vi "Data_Aquisition_cRIO4.vi"() -> ()   [LabVIEW 2016]
uses:
  <vilib>/Platform/TimedLoop/XDataNode/timing_clust.ctl
  <vilib>/Platform/TimedLoop/XDataNode/nitl_modes.ctl
  <vilib>/Platform/TimedLoop/XDataNode/wakeup.ctl
  <vilib>/Utility/file.llb/Write Delimited Spreadsheet (string).vi
  <vilib>/Platform/TimedLoop/XDataNode/loadnilvce.vi
  <vilib>/Utility/file.llb/Write Delimited Spreadsheet (DBL).vi
  <vilib>/Platform/TimedLoop/XDataNode/XDataNode.xnode
  <vilib>/Platform/TimedLoop/XDataNode/XDNodeRunTimeDep.lvlib
panel:
  in  "Mod 2 Labels":string[][](array[string])=[["M2AO0", "M2AO1"], ["Air", "N2"]]
  in  "Mod 1 Labels":string[][](array[string])=[["M1DO0", "M1DO1", "M1DO2", "M1DO3", "M1DO4", "M1DO5", "M1DO6"], ["Inf", "Eff", "Acid", "Base", "Media", "Air", "Release"]]
  in  "Mod 3 Labels":string[][](array[string])=[["M3AI0", "M3AI1", "M3AI2", "M3AI3", "M3AI4"], ["pH", "DO", "Air", "N2", "Off"]]
  out "data":dbl[][](array[numeric])=[[8.0, 29.0, 2018.0, 14421397.0, 0.0, 0.0, 0.0, 0.0, 0.0, 1.0, 0.0, 0.003999706016, 0.003999847522999999, 0.012958363706999999, 0.004113970148, -1.9721429999999986e-06, 0.0039692390630000005, 0.003999705047], [8.0, 29.0, 2018.0, 14421638.0, 0.0, 0.0, 0.0, 0.0, 0.0, 1.0, 0.0, 0.003999706016, 0.003999847522999999, 0.012891145231999999, 0.004107738319, -1.6440880000000006e-06, 0.003968582989, 0.004000361167]]
  out "headers":string[][](array[string])=[["Month", "Day", "Year", "Time", "M1DO0", "M1DO1", "M1DO2", "M1DO3", "M1DO4", "M1DO5", "M1DO6", "M2DO0", "M2DO1", "M3DO0", "M3DO1", "M3DO2", "M3DO3", "M3DO4"], ["Month", "Day", "Year", "Time", "Inf", "Eff", "Acid", "Base", "Media", "Air", "Release", "Air", "N2", "pH", "DO", "Air", "N2", "Off"]]
  out "Time":string="144216.38"
  out "Date":string="08292018"
  in  "Buffer Size":i32=6
  out "Saving?":bool=TRUE
  out "new file path (Not A Path if cancelled)":path=path "u:/_08292018_140859.csv"
  in  "File Name:":string
  out "error out":errorcluster
  out "iter number":i32=34
  in  "stop":bool
  in  "error in":errorcluster
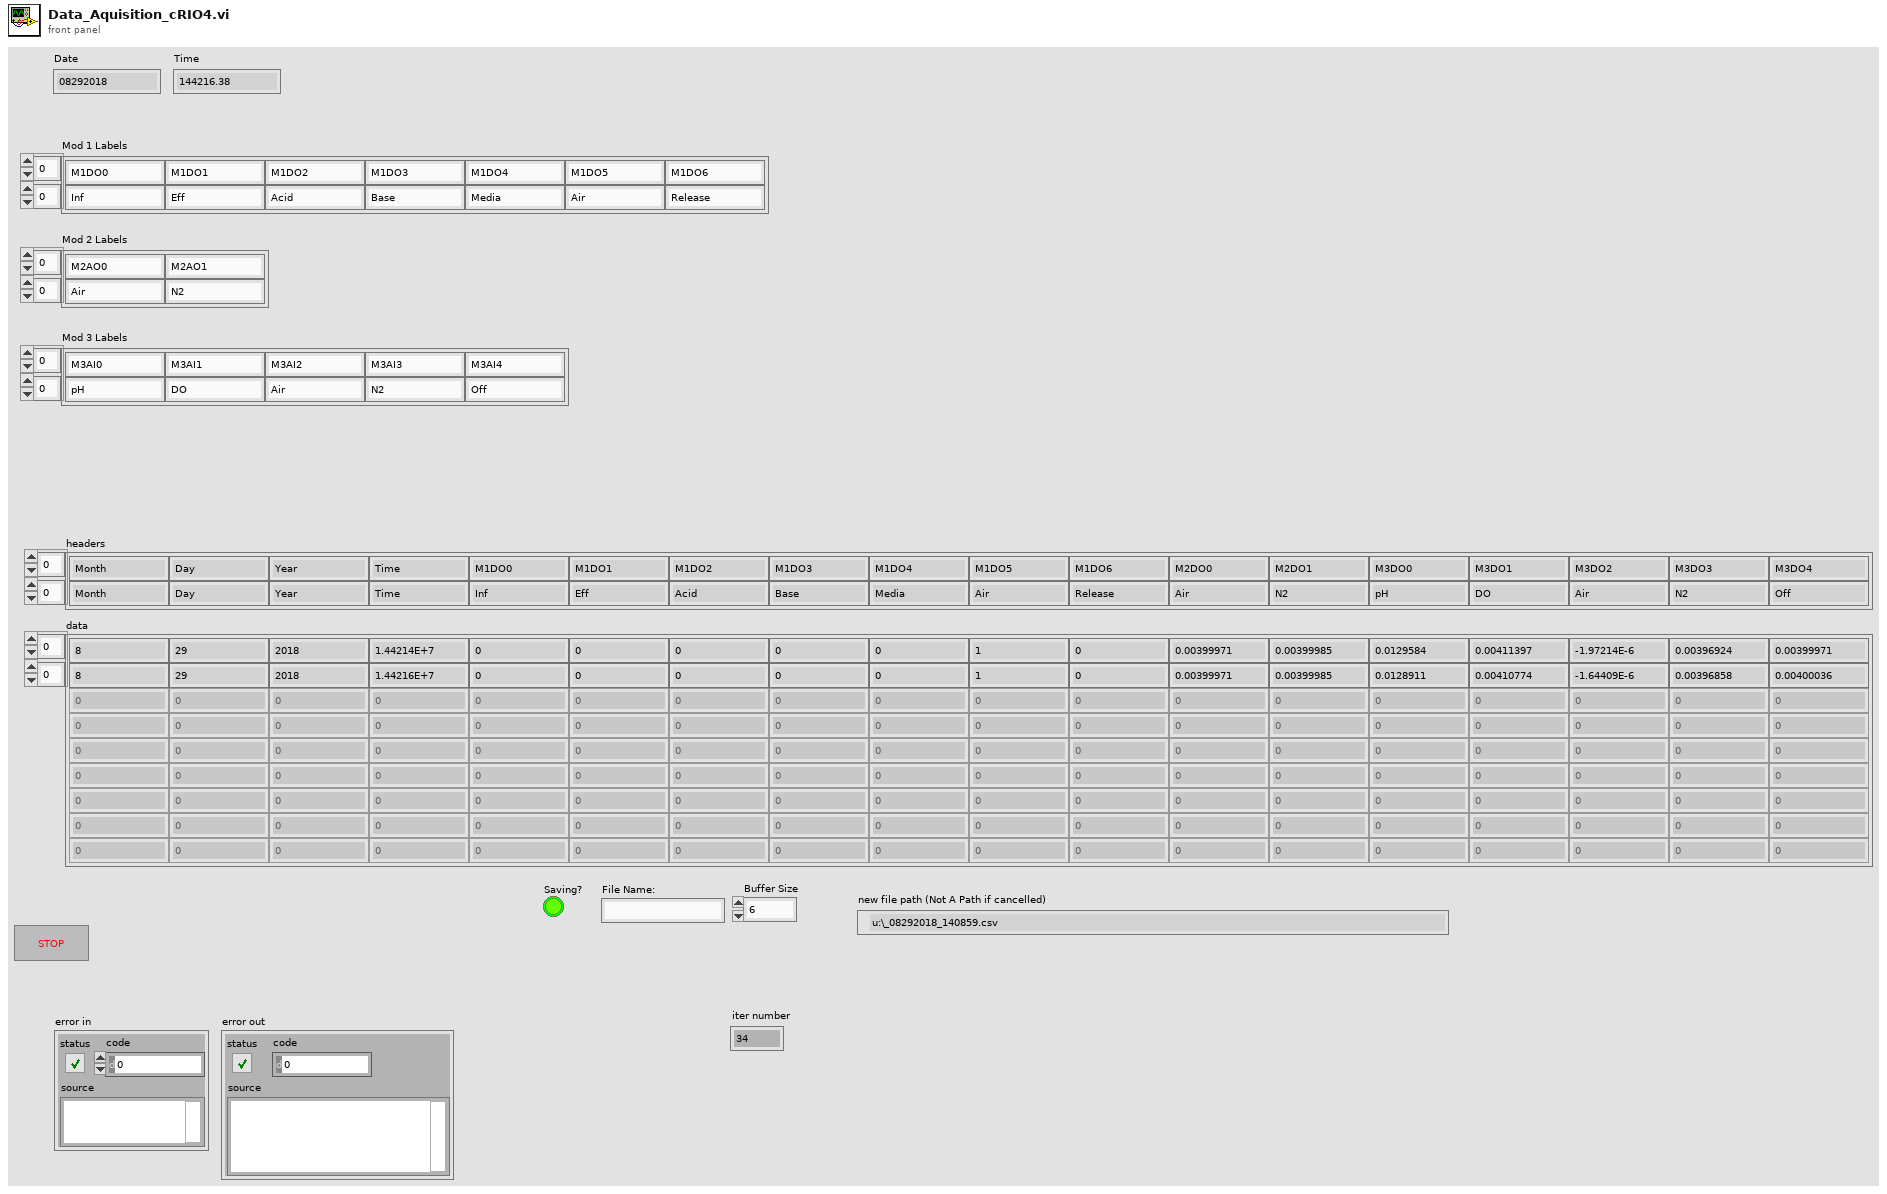
[diagram p1: front panel]
types:
  T1 = typedef "XDNodeRunTimeDep.lvlib/timing_clust.ctl" = cluster{"Expected End [f-1]":u64, "Actual End [f-1]":u64, "Finished Late? [f-1]":bool, "Expected End [i-1]":u64, "Actual End [i-1]":u64, "Finished Late? [i-1]":bool, "Expected Start [i]":u64, "Actual Start [i]":u64, "Expected Start [f]":u64, "Actual Start [f]":u64, "Source Name":string, "Structure Name":string, "Period":i64, "Deadline":i64, "Offset":i64, "Start":i64, "Priority":i32, "Timeout":i32, "Mode":T2, "Wakeup Reason":T3, "Error":errorcluster, "Source Type":string, "Secondary Source Type":string, "Global End Time":u64, "Global Start Time":u64, "Frame Duration":u64, "Iteration Duration":u64, "Assigned CPU":i32, "I/O Scan Engine Mode":u32}
  T2 = typedef "XDNodeRunTimeDep.lvlib/nitl_modes.ctl" = enum32{"No Change", "Process missed periods, maintain original phase", "Discard missed periods, maintain original phase", "Process missed periods, ignore original phase", "Discard missed periods, ignore original phase"}
  T3 = typedef "XDNodeRunTimeDep.lvlib/wakeup.ctl" = enum32{"Normal", "Aborted", "Asynchronous wakeup", "Timing source error", "Timed loop error", "Timeout"}
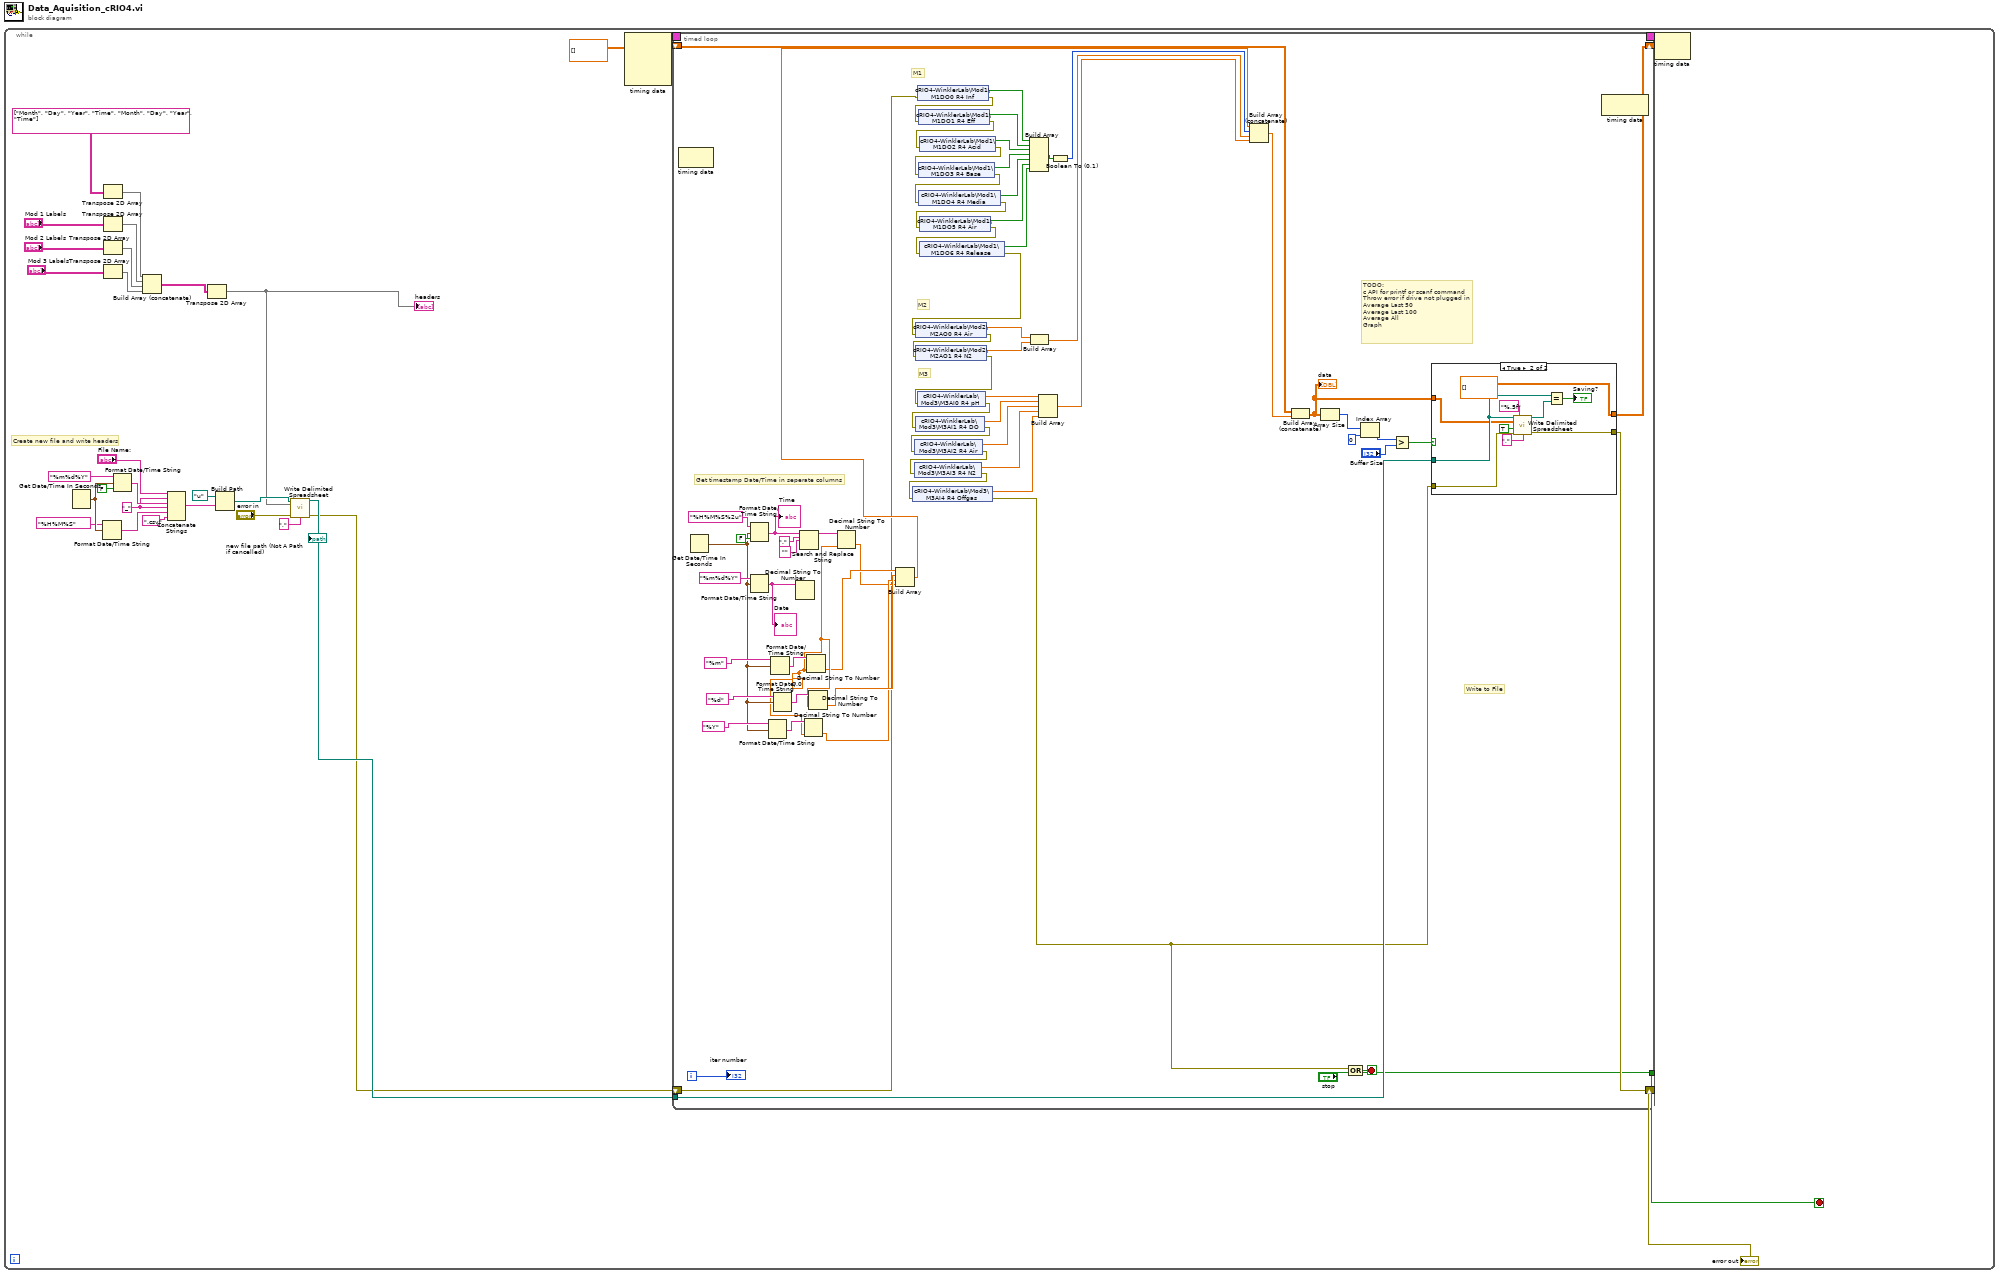
[diagram p0: block diagram]
diagram:
  n1 = while {
    stop <- w16 stop-if-true
    w19 = "_" ("string")
    # "Create new file and write headers"
    n2 = Get Date/Time In Seconds() -> (seconds since 1Jan1904=w24:timestamp)
    n3 = Format Date/Time String(time format string (%c)="%H%M%S", seconds (now)=w24) -> (date/time string=w18:string)  [unwired: 1 in]
    n4 = Transpose 2D Array(2D array=string[][] [["Month", "Day", "Year", "Time"], ["Month", "Day", "Year", "Time"]]) -> (transposed array=w8:string[][])
    n5 = Transpose 2D Array(2D array="Mod 1 Labels") -> (transposed array=w7:string[][])
    n6 = Transpose 2D Array(2D array="Mod 2 Labels") -> (transposed array=w6:string[][])
    n7 = Transpose 2D Array(2D array="Mod 3 Labels") -> (transposed array=w5:string[][])
    n8 = Format Date/Time String(time format string (%c)="%m%d%Y", seconds (now)=w24, UTC format=FALSE) -> (date/time string=w20:string)
    n9 = Build Array (concatenate)(w8, w7, w6, w5) -> (w10:string[][])
    n10 = Concatenate Strings("File Name:", w19, w20, w19, w18, ".csv" ("string")) -> (w17:string)
    n11 = Transpose 2D Array(2D array=w10) -> (transposed array=w4:string[][])
    "headers" <- w4
    n12 = Build Path(base path=path "u:/" ("Save to:"), name or relative path=w17) -> (appended path=w27:path)
    n13 = call-poly <vilib>:"Write Delimited Spreadsheet.vi"("file path (dialog if empty)"=w27, "2D data"=w4, "error in (no error)"="error in", "delimiter (\\t)"="," ("delimiter (\\t)")) -> ("new file path (Not A Path if cancelled)"=w31:path, "error out"=w30:errorcluster)  [unwired: 10 in]
    "new file path (Not A Path if cancelled)" <- w31
    n14 = node-c288() -> (w15:T1)  [unwired: 4 in]
    n15 = timed-loop {
      tunnel: w31 -> [w92]
      shift-right: [w78] -> _
      shift-left: dbl[][] [] -> [w97]
      shift-right: [w90] -> w11
      shift-left: w30 -> [w45]
      tunnel: ["stop"] -> w16
      timing: w15 -> [_]
      timing-out: [_] -> w14
      i -> [w98]
      stop <- w99 stop-if-true
      w69 = 0.0
      # "M3"
      # "M2"
      # "M1"
      # "TODO: \nc API for printf or scanf command\nThrow error if drive not plugged in\nAverage Last 50\nAverage Last 100\nAverage All\nGraph"
      # "Write to File"
      # "Get timestamp Date/Time in seperate columns"
      n16 = node-c288() -> ()  [unwired: 1 in, 1 out]
      n17 = Get Date/Time In Seconds() -> (seconds since 1Jan1904=w70:timestamp)
      n18 = Format Date/Time String(time format string (%c)="%H%M%S%2u", seconds (now)=w70, UTC format=FALSE) -> (date/time string=w85:string)
      "Time" <- w85
      n19 = Format Date/Time String(time format string (%c)="%m%d%Y", seconds (now)=w70) -> (date/time string=w82:string)  [unwired: 1 in]
      "Date" <- w82
      n20 = Format Date/Time String(time format string (%c)="%Y", seconds (now)=w70) -> (date/time string=w71:string)  [unwired: 1 in]
      n21 = Format Date/Time String(time format string (%c)="%m", seconds (now)=w70) -> (date/time string=w75:string)  [unwired: 1 in]
      n22 = Format Date/Time String(time format string (%c)="%d", seconds (now)=w70) -> (date/time string=w73:string)  [unwired: 1 in]
      n23 = Decimal String To Number(string=w82) -> ()  [unwired: 2 in, 2 out]
      n24 = Search and Replace String(input string=w85, search string=".", replace string="") -> (result string=w84:string)  [unwired: 5 in, 3 out]
      n25 = Decimal String To Number(string=w71, default (0L)=w69) -> (number=w66:dbl)  [unwired: 1 in, 1 out]
      n26 = Decimal String To Number(string=w75, default (0L)=w69) -> (number=w68:dbl)  [unwired: 1 in, 1 out]
      n27 = Decimal String To Number(string=w73, default (0L)=w69) -> (number=w67:dbl)  [unwired: 1 in, 1 out]
      n28 = Decimal String To Number(string=w84, default (0L)=w69) -> (number=w65:dbl)  [unwired: 1 in, 1 out]
      n29 = Build Array(w68, w67, w66, w65) -> (w58:dbl[])
      n30 = shared-variable "cRIO4-WinklerLab\\Mod1\\M1DO0 R4 Inf"(error in=w45) -> (w38:bool, error out=w44:errorcluster)
      n31 = shared-variable "cRIO4-WinklerLab\\Mod1\\M1DO1 R4 Eff"(error in=w44) -> (w37:bool, error out=w43:errorcluster)
      n32 = shared-variable "cRIO4-WinklerLab\\Mod1\\M1DO2 R4 Acid"(error in=w43) -> (w36:bool, error out=w42:errorcluster)
      n33 = shared-variable "cRIO4-WinklerLab\\Mod1\\M1DO3 R4 Base"(error in=w42) -> (w35:bool, error out=w41:errorcluster)
      n34 = shared-variable "cRIO4-WinklerLab\\Mod1\\M1DO4 R4 Media"(error in=w41) -> (w34:bool, error out=w40:errorcluster)
      n35 = shared-variable "cRIO4-WinklerLab\\Mod1\\M1DO5 R4 Air"(error in=w40) -> (w33:bool, error out=w39:errorcluster)
      n36 = shared-variable "cRIO4-WinklerLab\\Mod1\\M1DO6 R4 Release"(error in=w39) -> (w32:bool, error out=w46:errorcluster)
      n37 = shared-variable "cRIO4-WinklerLab\\Mod2\\M2AO0 R4 Air"(error in=w46) -> (w63:dbl, error out=w64:errorcluster)
      n38 = shared-variable "cRIO4-WinklerLab\\Mod2\\M2AO1 R4 N2"(error in=w64) -> (w62:dbl, error out=w47:errorcluster)
      n39 = shared-variable "cRIO4-WinklerLab\\Mod3\\M3AI0 R4 pH"(error in=w47) -> (w52:dbl, error out=w54:errorcluster)
      n40 = shared-variable "cRIO4-WinklerLab\\Mod3\\M3AI1 R4 DO"(error in=w54) -> (w51:dbl, error out=w53:errorcluster)
      n41 = shared-variable "cRIO4-WinklerLab\\Mod3\\M3AI2 R4 Air"(error in=w53) -> (w50:dbl, error out=w55:errorcluster)
      n42 = shared-variable "cRIO4-WinklerLab\\Mod3\\M3AI3 R4 N2"(error in=w55) -> (w49:dbl, error out=w56:errorcluster)
      n43 = shared-variable "cRIO4-WinklerLab\\Mod3\\M3AI4 R4 Offgas"(error in=w56) -> (w48:dbl, error out=w57:errorcluster)
      n44 = Build Array(w38, w37, w36, w35, w34, w33, w32) -> (w61:bool[])
      n45 = Build Array(w63, w62) -> (w60:dbl[])
      n46 = Build Array(w52, w51, w50, w49, w48) -> (w80:dbl[])
      n47 = Boolean To (0,1)(Boolean=w61) -> (0, 1=w59:i16[])
      n48 = Build Array (concatenate)(w58, w59, w60, w80) -> (w79:dbl[])
      n49 = Build Array (concatenate)(w97, w79) -> (w77:dbl[][])
      "data" <- w77
      n50 = Array Size(array=w77) -> (size(s)=w96:i32[])
      n51 = Compound Arithmetic op=OR(w57, "stop") -> (w99:bool)
      n52 = Index Array(array=w96, index=0) -> (element=w94:i32)
      n53 = Greater?(x=w94, y="Buffer Size") -> (0:w93:bool)
      n54 = case shown="True" w93 {
        tunnel: w77 -> [w103 w104]
        tunnel: w92 -> [_ w111]
        tunnel: [w103 dbl[][] []] -> w78
        tunnel: [w102 w110] -> w90
        tunnel: w57 -> [w102 w105]
        frame False {
        }
        frame True {
          n55 = call-poly <vilib>:"Write Delimited Spreadsheet.vi"("file path (dialog if empty)"=w111, "format (%.3f)"="%.5f", "2D data"=w104, "append to file? (new file:F)"=TRUE, "error in (no error)"=w105, "delimiter (\\t)"="," ("delimiter (\\t)")) -> ("new file path (Not A Path if cancelled)"=w112:path, "error out"=w110:errorcluster)  [unwired: 8 in]
          n56 = Equal?(x=w111, y=w112) -> (x = y?=→"Saving?":bool)
        }
      }
      n57 = node-c288() -> ()  [unwired: 1 in, 1 out]
      "iter number" <- w98
    }
    "error out" <- w11
    n58 = node-c288(w14) -> ()  [unwired: 1 out]
  }
